vi "stringConvertToDate2.vi"(1 "input_str_yymmdd":string="2015/11/23 8:14:18") -> (0 "show_date":timestamp)   [LabVIEW 2011]
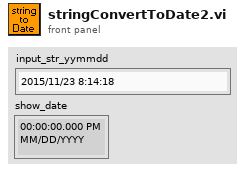
[diagram p1: front panel]
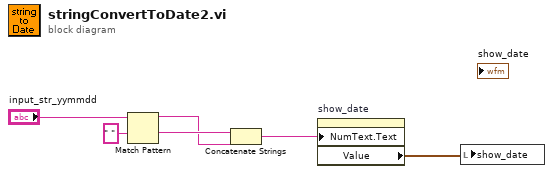
[diagram p0: block diagram]
diagram:
  n1 = Match Pattern(string="input_str_yymmdd", regular expression=" " ("正则表达式")) -> (before substring=w2:string, after substring=w3:string)  [unwired: 1 in, 2 out]
  n2 = Concatenate Strings(w3, w2) -> (w1:string)
  n3 = property on="show_date" class="AbsTime (严格)"("NumText.Text"=w1) -> ("Value"=w6:timestamp)  [unwired: 2 in, 2 out]
  n4 = local write "show_date"(w6) -> ()
